vi "Configure Active Phase.vi"(0 "VISA resource name":refnum<visa-resource-name>, 5 "Output Phase(s) (3-Phase)":u16(ring)=3 items=["1-Phase"=1, "3-Phase"=3], 7 "Enable Coupling (Enabled)":bool=TRUE, 9 "Active Phase (1:Phase 1)":i32(ring)=1 items=["Phase 1"=1, "Phase 2"=2, "Phase 3"=3], 11 "error in (no error)":errorcluster) -> (4 "VISA resource name out":refnum<visa-resource-name>, 15 "error out":errorcluster)   [LabVIEW 2013, in "California Instruments iX Series.lvlib"]
doc: "Configures the three phase output capability of the AC Power Source. \n\n<b>Note:</b>\nThis VI does not support single phase output models. Single phase units always operate on Phase A only."
uses:
  California Instruments iX Series.lvlib
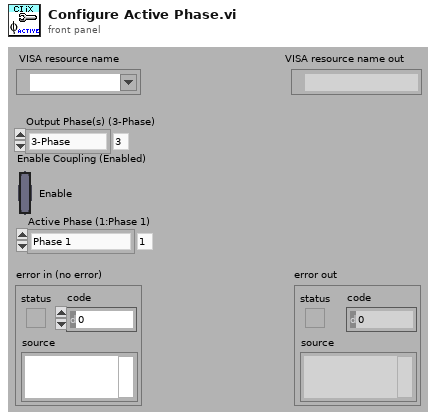
[diagram p1: front panel]
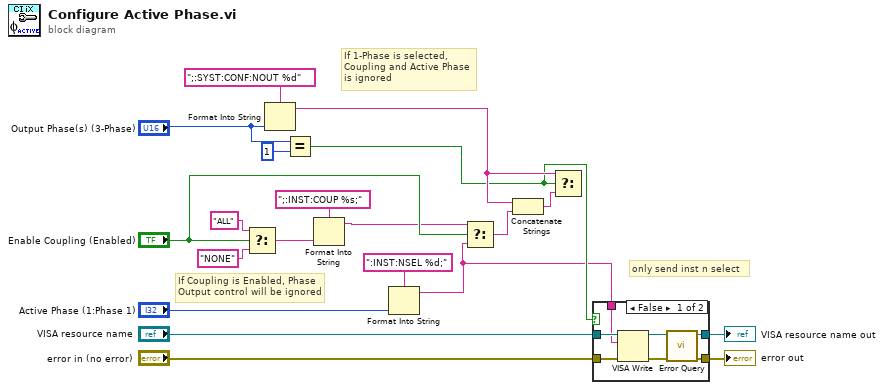
[diagram p0: block diagram]
diagram:
  # "only send inst n select"
  # "If 1-Phase is selected, Coupling and Active Phase is ignored"
  # "If Coupling is Enabled, Phase Output control will be ignored"
  n1 = Select(t="ALL", s="Enable Coupling (Enabled)", f="NONE") -> (s? t:f=w13:string)
  n2 = Format Into String(format string=";:SYST:CONF:NOUT %d", "Output Phase(s) (3-Phase)") -> (resulting string=w5:string)  [unwired: 2 in, 1 out]
  n3 = Equal?(x="Output Phase(s) (3-Phase)", y=u16 1) -> (x = y?=w2:bool)
  n4 = Format Into String(format string=";:INST:COUP %s;", w13) -> (resulting string=w9:string)  [unwired: 2 in, 1 out]
  n5 = Format Into String(format string=":INST:NSEL %d;", "Active Phase (1:Phase 1)") -> (resulting string=w1:string)  [unwired: 2 in, 1 out]
  n6 = Select(t=w9, s="Enable Coupling (Enabled)", f=w1) -> (s? t:f=w4:string)
  n7 = Concatenate Strings(w5, w4) -> (w3:string)
  n8 = Select(t=w5, s=w2, f=w3) -> ()  [unwired: 1 out]
  n9 = case shown="False" w2 {
    tunnel: [w27 w28] -> w20
    tunnel: [w26 w29] -> w19
    tunnel: "VISA resource name" -> [w23 w29]
    tunnel: "error in (no error)" -> [w22 w28]
    tunnel: w1 -> [w21 _]
    frame False {
      n10 = VISA Write(VISA resource name=w23, write buffer=w21, error in (no error)=w22) -> (VISA resource name out=w25:refnum<visa-resource-name>, error out=w24:errorcluster)  [unwired: 1 out]
      n11 = call "Error Query.vi"("error in (no error)"=w24, "VISA resource name"=w25) -> ("error out"=w27:errorcluster, "VISA resource name out"=w26:refnum<visa-resource-name>)  [unwired: 6 in, 2 out]
    }
    frame True {
    }
  }
  "error out" <- w20
  "VISA resource name out" <- w19
